vi "Database.vi"(8 "error in":errorcluster, 10 "Action":T1, 11 "User Input":string) -> (0 "error out":errorcluster, 3 "Name":string)   [LabVIEW 2019]
uses:
  ATM Action.ctl
  SubVI.lvlib
panel:
  out "Money Out":string
  in  "Money In":string
  out "Done":bool
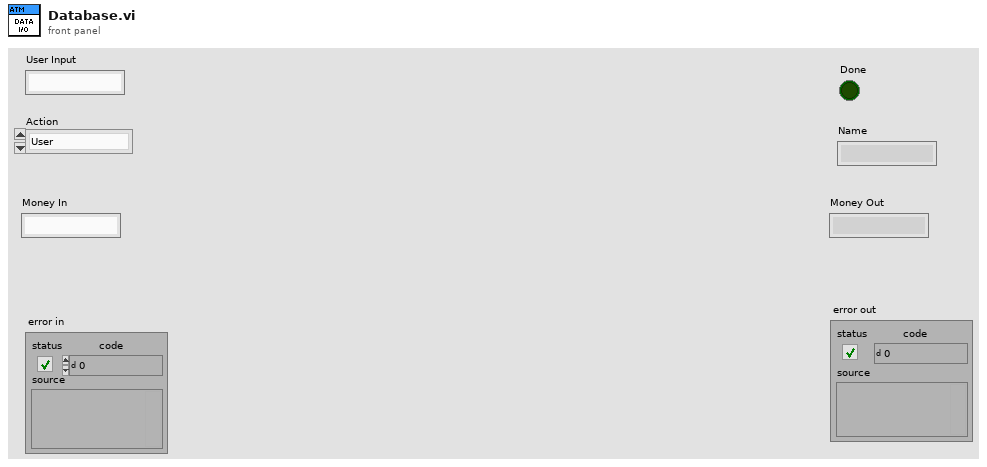
[diagram p1: front panel]
types:
  T1 = typedef "ATM Action.ctl" = enum16{"User", "Deposit", "Withdraw"}
  T2 = cluster{"Account":string, "First":string, "Last":string, "Money":string}[]
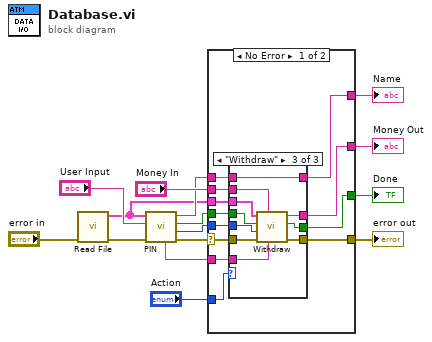
[diagram p0: block diagram]
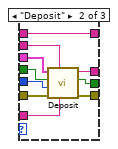
[diagram p3: hidden frame]
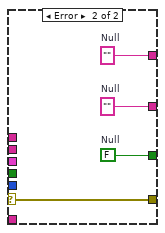
[diagram p4: hidden frame]
diagram:
  n1 = call "Read File.vi"("error in (no error)"="error in") -> ("error out"=w8:errorcluster, "Account Details"=w1:T2)  [unwired: 9 in]
  n2 = call "PIN.vi"("error in (no error)"=w8, "User Input"="User Input", "Account Details"=w1) -> ("error out"=w7:errorcluster, "Index"=w2:i32, "Valid"=w3:bool, "Name"=w5:string, "Money"=w4:string)  [unwired: 4 in]
  n3 = case shown="No Error" w7 {
    selector: w7 -> [w25 w55]
    tunnel: "Action" -> [w27 _]
    tunnel: "Money In" -> [w26 _]
    tunnel: [w17 w53] -> w13
    tunnel: [w16 w55] -> w14
    tunnel: [w24 w54] -> w12
    tunnel: [w23 w52] -> w10
    tunnel: w5 -> [w18 _]
    tunnel: w4 -> [w21 _]
    tunnel: w3 -> [w20 _]
    tunnel: w2 -> [w19 _]
    tunnel: w1 -> [w22 _]
    frame No Error {
      n4 = case shown="\"Withdraw\"" w27 {
        tunnel: w26 -> [_ w40 w51]
        tunnel: w25 -> [w28 w38 w43]
        tunnel: [w29 w39 w49] -> w24
        tunnel: [w30 w41 w50] -> w23
        tunnel: w22 -> [_ w37 w48]
        tunnel: w21 -> [w30 w34 w47]
        tunnel: w20 -> [w29 w36 w46]
        tunnel: w19 -> [_ w35 w45]
        tunnel: w18 -> [w31 w33 w44]
        tunnel: [w31 w33 w44] -> w17
        tunnel: [w28 w32 w42] -> w16
        frame "User" {
        }
        frame "Deposit" {
          n5 = call "Deposit.vi"("Money DB"=w34, "Money In"=w40, "error in (no error)"=w38, "Index"=w35, "Valid"=w36, "Account Details"=w37) -> ("error out"=w32:errorcluster, "Done"=w39:bool, "Money Out"=w41:string)  [unwired: 3 in]
        }
        frame "Withdraw" {
          n6 = call "Withdraw.vi"("Money DB"=w47, "Money In"=w51, "error in (no error)"=w43, "Index"=w45, "Valid"=w46, "Account Details"=w48) -> ("error out"=w42:errorcluster, "Done?"=w49:bool, "Money Out"=w50:string)  [unwired: 3 in]
        }
      }
    }
    frame Error {
      w52 = ""  # Null
      w53 = ""  # Null
      w54 = FALSE  # Null
    }
  }
  "Name" <- w13
  "Done" <- w12
  "error out" <- w14
  "Money Out" <- w10
